vi "Measure Current and Burst Waveform.vi"() -> ()   [LabVIEW 2021]
uses:
  <instrlib>/niDCPower/nidcpower.llb/niDCPower Source Mode.ctl
  <instrlib>/niDCPower/nidcpower.llb/niDCPower Wait For Event - Event.ctl
  <instrlib>/niDCPower/nidcpower.llb/niDCPower Output Function.ctl
  <instrlib>/niDMM/nidmm.llb/niDMM Function.ctl
  <instrlib>/niDMM/nidmm.llb/niDMM Configure Measurement Digits.vi
panel:
  in  "Fgen Channel":string
  in  "Waveform":T1(ring)=enum."Noise"
  in  "Frequency":dbl=6.0
  in  "Amplitude":dbl=6.0
  in  "Fgen":refnum<k15>
  out "Actual Duration":dbl
  in  "duration":dbl
  in  "Load DMM":refnum<k15>="Dev1"
  out "Current in DMM":dbl caption="Current Measurement"
  in  "Resolution in Digits":dbl(ring)=5.5 items=["3 1/2"=3.5, "4 1/2"=4.5, "5 1/2"=5.5, "6 1/2"=6.5, "7 1/2"=7.5]
  out "Signal Out of Range":bool
  in  "Range (Amps)":dbl=0.2 format="%.2p"
  in  "error in":errorcluster
  out "error out":errorcluster
  out "Voltage Measurement":dbl
  out "Current Measurement":dbl
  in  "Voltage Limit Range":dbl=6.0 format="%.5p"
  in  "Current Level Range":dbl=0.01 format="%.3p"
  in  "Voltage Limit":dbl=2.0 format="%.5p"
  in  "Current Level":dbl=0.01 format="%.3p"
  in  "Load SMU Channel":string="0"
  in  "Load SMUs":refnum<k15>="Dev1" caption="Load SMU"
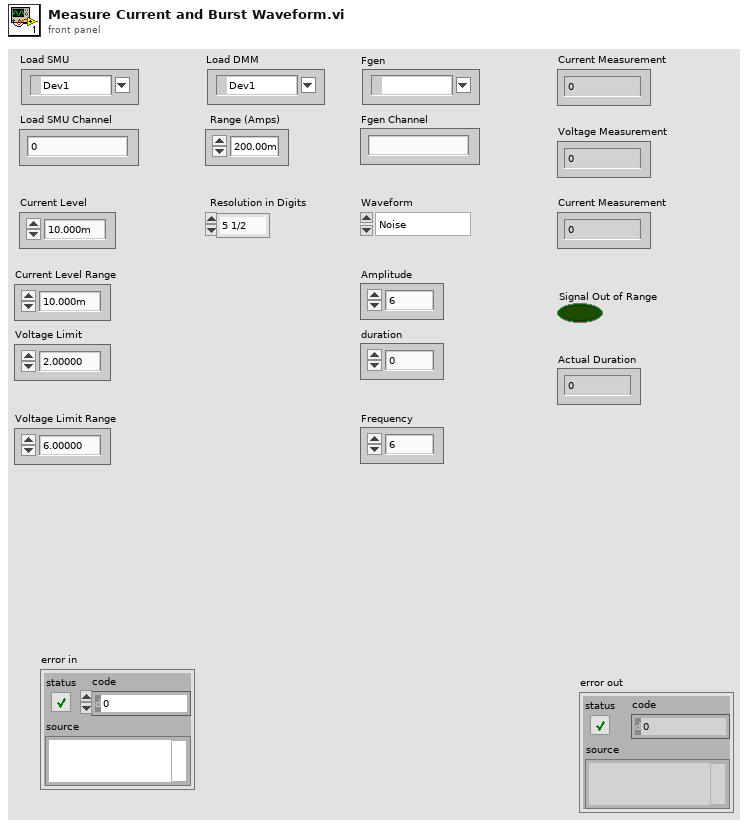
[diagram p1: front panel]
types:
  T1 = enum32{"Sine", "Square", "Triangle", "Ramp Up", "Ramp Down", "DC", "Noise", "User"}
  T2 = typedef "niDMM Function.ctl" = enum16{"DC Volts", "AC Volts", "DC Current", "AC Current", "2-wire Resistance", "4-wire Resistance", "Diode", "Frequency", "Period", "AC Volts DC Coupled", "Capacitance", "Inductance", "Temperature"}
  T3 = typedef "niDCPower Output Function.ctl" = i32
  T4 = typedef "niDCPower Wait For Event - Event.ctl" = i32
  T5 = typedef "niDCPower Source Mode.ctl" = i32
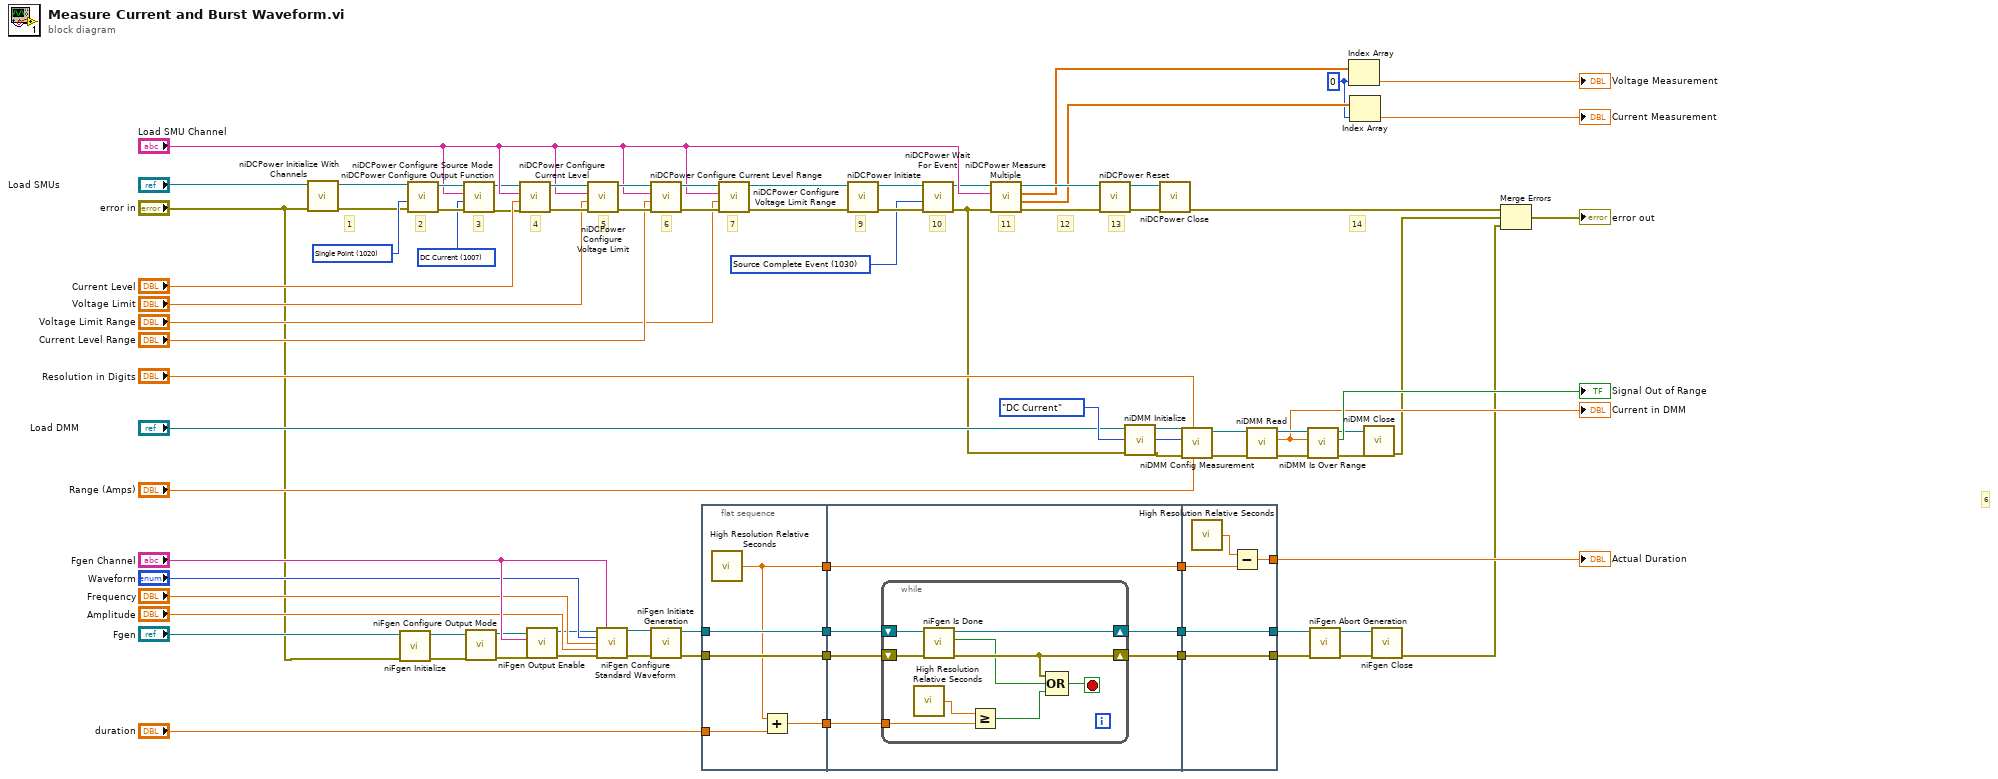
[diagram p0: block diagram]
diagram:
  w55 = T3 1007 items=["DC Voltage"=1006, "DC Current"=1007, "Pulse Voltage"=1049, "Pulse Current"=1050] ("output function")
  w58 = T4 1030 items=["Source Complete Event"=1030, "Measure Complete Event"=1031, "Sequence Iteration Complete Event"=1032, "Sequence Engine Done Event"=1033] ("event")
  w67 = 0 ("index")
  w77 = T5 1020 items=["Single Point"=1020, "Sequence"=1021] ("source mode")
  # "6"
  # "14"
  # "11"
  # "10"
  # "7"
  # "6"
  # "2"
  # "3"
  # "12"
  # "13"
  # "9"
  # "5"
  # "4"
  # "1"
  n1 = call <instrlib>:"niDCPower Initialize With Channels.vi"("error in (no error)"="error in", "resource name"="Load SMUs") -> ("error out"=w41:errorcluster, "instrument handle out"=w42:refnum<k15>)  [unwired: 8 in]
  n2 = call <instrlib>:"niFgen Initialize.vi"("error in (no error)"="error in", "Resource Name"="Fgen") -> ("error out"=w12:errorcluster, "Instrument Handle Out"=w9:refnum<k15>)  [unwired: 8 in]
  n3 = call <instrlib>:"niDCPower Configure Source Mode.vi"("error in (no error)"=w41, "source mode"=w77, "instrument handle"=w42) -> ("error out"=w79:errorcluster, "instrument handle out"=w78:refnum<k15>)  [unwired: 7 out]
  n4 = call <instrlib>:"niDCPower Configure Output Function.vi"("error in (no error)"=w79, "output function"=w55, "channel name"="Load SMU Channel", "instrument handle"=w78) -> ("error out"=w57:errorcluster, "instrument handle out"=w56:refnum<k15>)  [unwired: 6 out]
  n5 = call <instrlib>:"niFgen Configure Output Mode.vi"("error in (no error)"=w12, "Instrument Handle"=w9) -> ("error out"=w22:errorcluster, "Instrument Handle Out"=w13:refnum<k15>)  [unwired: 7 in]
  n6 = call <instrlib>:"niDCPower Configure Current Level.vi"("error in (no error)"=w57, "current level"="Current Level", "channel name"="Load SMU Channel", "instrument handle"=w56) -> ("error out"=w82:errorcluster, "instrument handle out"=w83:refnum<k15>)  [unwired: 6 out]
  n7 = call <instrlib>:"niFgen Output Enable.vi"("error in (no error)"=w22, "Channel Name"="Fgen Channel", "Instrument Handle"=w13) -> ("error out"=w11:errorcluster, "Instrument Handle Out"=w14:refnum<k15>)  [unwired: 7 in]
  n8 = call <instrlib>:"niDCPower Configure Voltage Limit.vi"("error in (no error)"=w82, "voltage limit"="Voltage Limit", "channel name"="Load SMU Channel", "instrument handle"=w83) -> ("error out"=w76:errorcluster, "instrument handle out"=w75:refnum<k15>)  [unwired: 6 out]
  n9 = call <instrlib>:"niFgen Configure Standard Waveform.vi"("Instrument Handle"=w14, "Channel Name"="Fgen Channel", "Waveform"="Waveform", "Frequency"="Frequency", "Amplitude"="Amplitude", "error in (no error)"=w11) -> ("Instrument Handle Out"=w15:refnum<k15>, "error out"=w10:errorcluster)  [unwired: 8 in]
  n10 = call <instrlib>:"niDCPower Configure Current Level Range.vi"("error in (no error)"=w76, "current level range"="Current Level Range", "channel name"="Load SMU Channel", "instrument handle"=w75) -> ("error out"=w74:errorcluster, "instrument handle out"=w73:refnum<k15>)  [unwired: 6 out]
  n11 = call <instrlib>:"niFgen Initiate Generation.vi"("error in (no error)"=w10, "Instrument Handle"=w15) -> ("error out"=w18:errorcluster, "Instrument Handle Out"=w16:refnum<k15>)  [unwired: 8 in]
  n12 = flat-sequence {
    tunnel: w18 -> [w87]
    tunnel: w16 -> [w88]
    tunnel: [w88] -> w36
    tunnel: [w87] -> w35
    tunnel: [w86] -> w34
    tunnel: "duration" -> [w85]
    tunnel: [w84] -> w33
    tunnel: w36 -> [w94]
    tunnel: w35 -> [w92]
    tunnel: [w93] -> w32
    tunnel: [w91] -> w31
    tunnel: [w90] -> w30
    tunnel: w34 -> [w90]
    tunnel: w33 -> [w89]
    tunnel: [w107] -> w19
    tunnel: [w108] -> w17
    tunnel: w32 -> [w108]
    tunnel: w31 -> [w107]
    tunnel: w30 -> [w105]
    tunnel: [w104] -> w28
    frame #0 {
      n13 = call <vilib>:"High Resolution Relative Seconds.vi"() -> ("relative seconds"=w86:dbl)
      n14 = Add(x=w86, y=w85) -> (x+y=w84:dbl)
    }
    frame #1 {
      n15 = while {
        shift-right: [w102] -> w93
        shift-left: w94 -> [w103]
        shift-right: [w100] -> w91
        shift-left: w92 -> [w101]
        tunnel: w89 -> [w97]
        stop <- w99 stop-if-true
        n16 = call <vilib>:"High Resolution Relative Seconds.vi"() -> ("relative seconds"=w98:dbl)
        n17 = call <instrlib>:"niFgen Is Done.vi"("error in (no error)"=w101, "Instrument Handle"=w103) -> ("error out"=w100:errorcluster, "Done"=w95:bool, "Instrument Handle Out"=w102:refnum<k15>)  [unwired: 7 in]
        n18 = Greater Or Equal?(x=w98, y=w97) -> (x >= y?=w96:bool)
        n19 = Compound Arithmetic op=OR(w100, w95, w96) -> (w99:bool)
      }
    }
    frame #2 {
      n20 = call <vilib>:"High Resolution Relative Seconds.vi"() -> ("relative seconds"=w106:dbl)
      n21 = Subtract(x=w106, y=w105) -> (x-y=w104:dbl)
    }
  }
  n22 = call <instrlib>:"niDCPower Configure Voltage Limit Range.vi"("error in (no error)"=w74, "voltage limit range"="Voltage Limit Range", "channel name"="Load SMU Channel", "instrument handle"=w73) -> ("error out"=w63:errorcluster, "instrument handle out"=w64:refnum<k15>)  [unwired: 6 out]
  n23 = call <instrlib>:"niDCPower Initiate.vi"("error in (no error)"=w63, "instrument handle"=w64) -> ("error out"=w59:errorcluster, "instrument handle out"=w61:refnum<k15>)  [unwired: 2 in, 6 out]
  n24 = call <instrlib>:"niDCPower Wait For Event.vi"("error in (no error)"=w59, "event"=w58, "instrument handle"=w61) -> ("error out"=w38:errorcluster, "instrument handle out"=w60:refnum<k15>)  [unwired: 1 in, 6 out]
  n25 = call <instrlib>:"niDCPower Measure Multiple.vi"("error in (no error)"=w38, "channel name"="Load SMU Channel", "instrument handle"=w60) -> ("error out"=w46:errorcluster, "current measurements"=w68:dbl[], "voltage measurements"=w69:dbl[], "instrument handle out"=w70:refnum<k15>)  [unwired: 5 out]
  n26 = call <instrlib>:"niDCPower Reset.vi"("error in (no error)"=w46, "instrument handle"=w70) -> ("error out"=w5:errorcluster, "instrument handle out"=w6:refnum<k15>)  [unwired: 2 in, 6 out]
  n27 = call <instrlib>:"niDMM Initialize.vi"("error in (no error)"=w38, "Instrument Descriptor"="Load DMM") -> ("error out"=w37:errorcluster, "instrument handle out"=w39:refnum<k15>)  [unwired: 8 in]
  n28 = call <instrlib>:"niDCPower Close.vi"("error in (no error)"=w5, "instrument handle"=w6) -> ("error out"=w4:errorcluster)  [unwired: 9 in]
  n29 = call-poly <instrlib>:"niDMM Config Measurement.vi"("Range"="Range (Amps)", "Resolution in Digits"="Resolution in Digits", "error in (no error)"=w37, "Function"=niDMM_Function."DC Current", "instrument handle"=w39) -> ("error out"=w53:errorcluster, "instrument handle out"=w52:refnum<k15>)  [unwired: 5 in]
  n30 = call <instrlib>:"niDMM Read.vi"("error in (no error)"=w53, "instrument handle"=w52) -> ("error out"=w50:errorcluster, "Measurement"=w44:dbl, "instrument handle out"=w51:refnum<k15>)  [unwired: 7 in]
  "Current in DMM" <- w44
  n31 = call <instrlib>:"niDMM Is Over Range.vi"("error in (no error)"=w50, "Measurement"=w44, "instrument handle"=w51) -> ("error out"=w3:errorcluster, "Over Range?"=→"Signal Out of Range":bool, "instrument handle out"=w2:refnum<k15>)  [unwired: 6 in]
  n32 = call <instrlib>:"niFgen Abort Generation.vi"("error in (no error)"=w19, "Instrument Handle"=w17) -> ("error out"=w21:errorcluster, "Instrument Handle Out"=w20:refnum<k15>)  [unwired: 8 in]
  n33 = Index Array(array=w69, index=w67) -> (element=→"Voltage Measurement":dbl)
  n34 = Index Array(array=w68, index=w67) -> (element=→"Current Measurement":dbl)
  n35 = call <instrlib>:"niDMM Close.vi"("error in (no error)"=w3, "instrument handle"=w2) -> ("error out"=w1:errorcluster)  [unwired: 9 in]
  n36 = call <instrlib>:"niFgen Close.vi"("error in (no error)"=w21, "Instrument Handle"=w20) -> ("error out"=w7:errorcluster)  [unwired: 9 in]
  n37 = Merge Errors(w4, w1, w7) -> (→"error out":errorcluster)
  "Actual Duration" <- w28
